vi "temporary CE GUI main.vi"() -> ()   [LabVIEW 2020]
uses:
  Type definitions/CEmeter settings.ctl
  Utilities/Type definitions/Common properties.ctl
  General AC source/Type definitions/AC Source.ctl
  General AC source/Type definitions/AC Source type.ctl
  Utilities/Type definitions/Measurement properties.ctl
panel:
  in  "Settle down after AC source change (s)":dbl=5.0 format="%#_13g"
  in  "AC Source":T1={"AC Source type"=enum."Tektronix AFG3000 series", "VISA"="GPIB0::11::INSTR", "Ref. clock (Hz)"=10000000.0, "status ref"=refnum}
  out "Measurement points":i32
  out "Measurement frequencies":i32[](array[numeric]) caption="List of measurement frequencies"
  in  "Stop freuency (Hz)":i32=7000000 format="%#_7p"
  in  "Step freuency (Hz)":i32=200000 format="%#_7p"
  in  "Starting freuency":i32=1000 format="%#_7p"
  in  "Sampling frequency (Hz)":dbl=10000000.0 format="%#_13p"
  in  "Signal amplitude (V)":dbl=1.0 format="%#_13g"
  in  "AC source status":string
  in  "CEmeter settings":T3={"Common properties"={"Measurement status ref"=refnum, "TWM Status ref"=refnum, "Abort ref"=refnum, "Skip waiting ref"=refnum, "GNU Octave path"=path "C:/Program Files/GNU Octave/Octave-6.2.0/mingw64/bin", "TWM+QWTB path"=path "C:/Users/labina/Desktop/TWM-1.8.7.0-full/octprog", "lvlib path"=path "D:/martin/WAC/WACsw - github/control_software/Filter function meter/external libraries/GOLPI 0.7.3.1 source distribution LV 20.0 32 bit/lv_proc.dll", "TWM pipe"="\\\\.\\pipe\\TWM:server"}, "AC Source"={"AC Source type"=enum."Fluke 5XXX calibrator", "VISA"="", "Ref. clock (Hz)"=0.0, "status ref"=refnum}, "Measurement properties"={"Signal frequencies (Hz)"=[1000.0], "Signal amplitudes (V)"=[0.707], "Sampling frequencies (Hz)"=[10000000.0], "Record lengths (multiples of periods)"=[10000.0], "TWM data directories"=[], "Calculate RMS from samples"=FALSE, "RMS algorithm"="TWM-WFFT"}, "Settle down after AC source change (s)"=1.0} {"Measurement properties"."Record lengths (multiples of periods)" format="%#_3p"; "Measurement properties"."Sampling frequencies (Hz)" format="%#_3p"; "Measurement properties"."Signal amplitudes (V)" format="%#_3p"; "Measurement properties"."Signal frequencies (Hz)" format="%#_3p"}
  in  "Divide frequency by this to\nget number of periods":i32=100
  out "freq / PFI0 A / PFI0 unc(A) / PFI1 A / PFI0 unc(A)":string[][](array[string])
  out "error out":errorcluster
  in  "Skip waiting":bool caption="Abort"
  in  "Abort":bool
  in  "TWM status":string
  in  "mesurement status":string
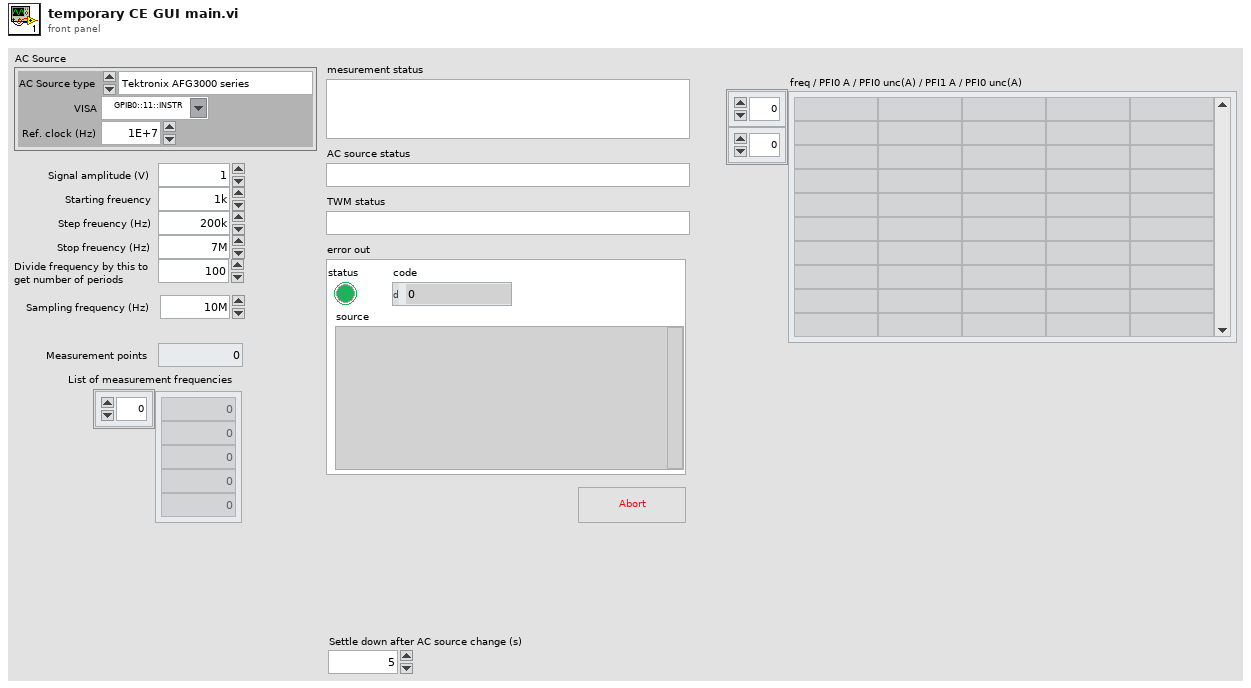
[diagram p1: front panel]
types:
  T1 = typedef "AC Source.ctl" = cluster{"AC Source type":T2, "VISA":refnum<visa-resource-name>, "Ref. clock (Hz)":dbl, "status ref":refnum<vi>}
  T2 = typedef "AC Source type.ctl" = enum16{"Fluke 5XXX calibrator", "Tektronix AFG3000 series", "dummy"}
  T3 = typedef "CEmeter settings.ctl" = cluster{"Common properties":T4, "AC Source":T1, "Measurement properties":T5, "Settle down after AC source change (s)":dbl}
  T4 = typedef "Common properties.ctl" = cluster{"Measurement status ref":refnum<vi>, "TWM Status ref":refnum<vi>, "Abort ref":refnum<vi>, "Skip waiting ref":refnum<vi>, "GNU Octave path":path, "TWM+QWTB path":path, "lvlib path":path, "TWM pipe":string}
  T5 = typedef "Measurement properties.ctl" = cluster{"Signal frequencies (Hz)":dbl[], "Signal amplitudes (V)":dbl[], "Sampling frequencies (Hz)":dbl[], "Record lengths (multiples of periods)":dbl[], "TWM data directories":string[], "Calculate RMS from samples":bool, "RMS algorithm":string}
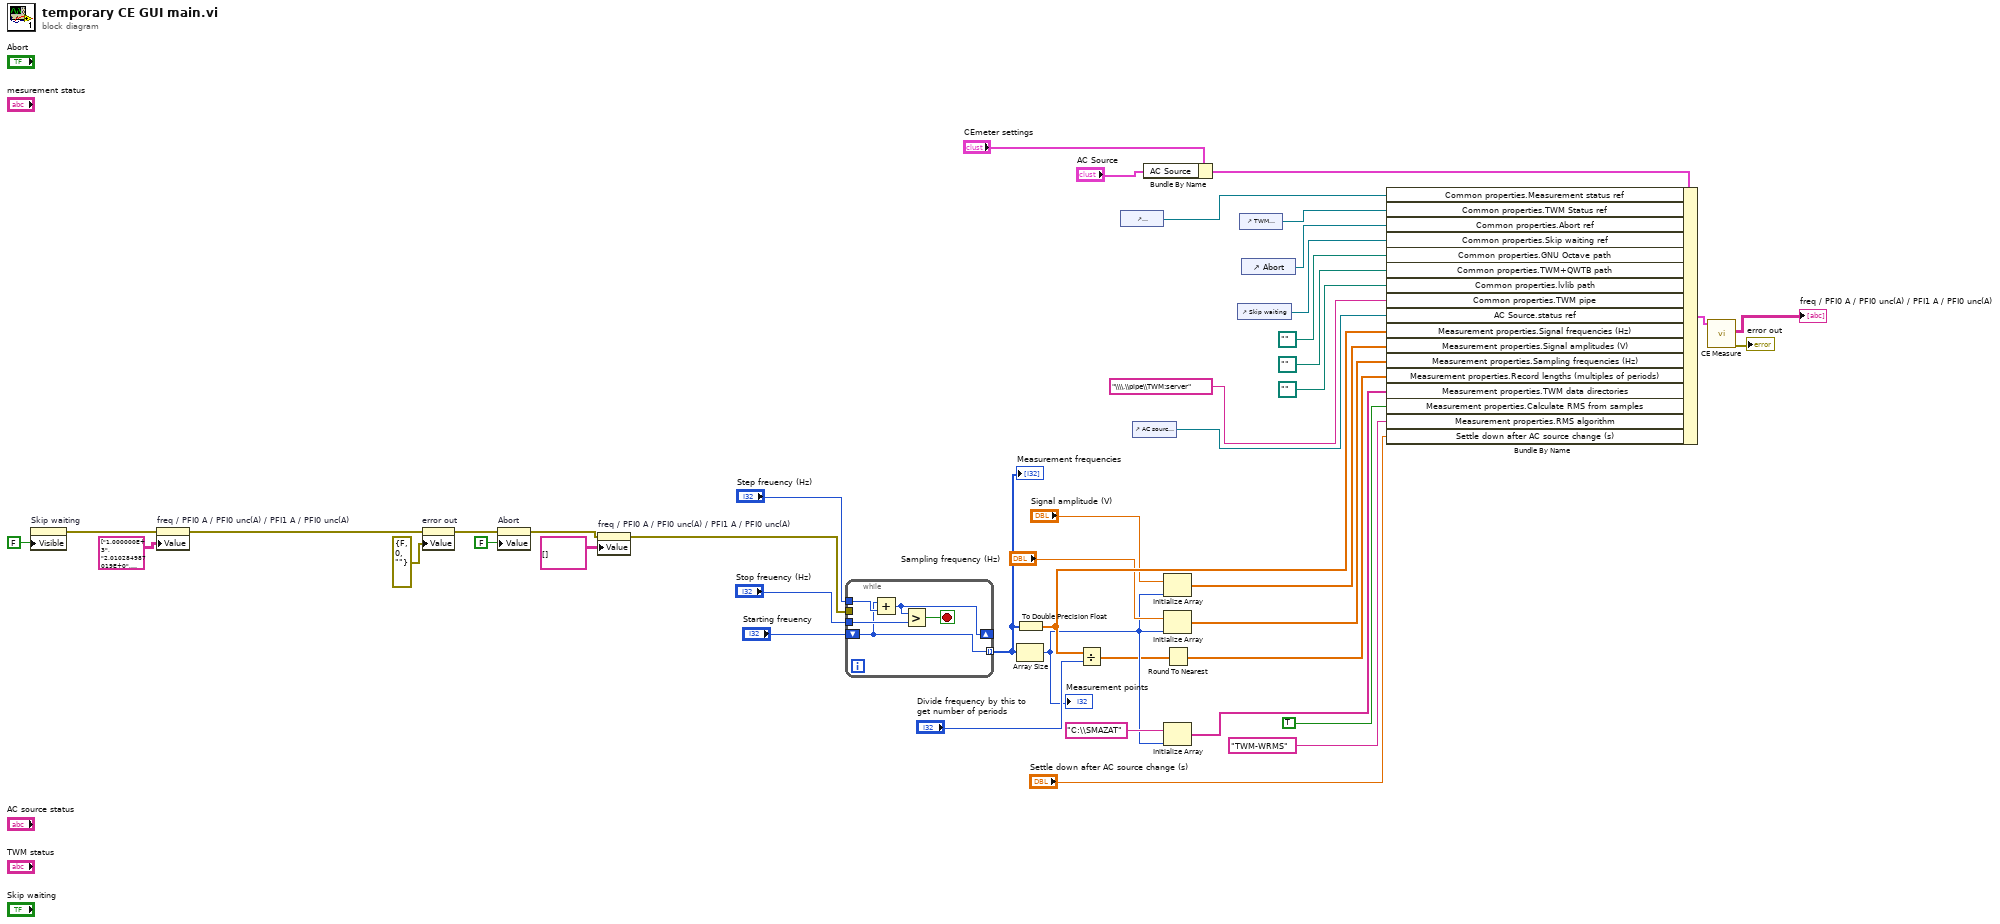
[diagram p0: block diagram]
diagram:
  n1 = property on="Skip waiting" class="Bool (strict)"("Visible"=FALSE) -> (error out=w5:errorcluster)  [unwired: 2 in, 1 out]
  n2 = property on="freq / PFI0 A / PFI0 unc(A) / PFI1 A / PFI0 unc(A)" class="Arr (strict)"(error in=w5, "Value"=string[][] [["1.000000E+3", "2.010284987019E+0", "0.000000000000E+0", "1.811642520698E+0", "0.000000000000E+0"], ["5.100000E+4", "2.013354055463E+0", "0.000000000000E+0", "1.812350667632E+0", "0.000000000000E+0"], ["1.010000E+5", "2.017282793567E+0", "0.000000000000E+0", "1.925150798750E+0", "0.000000000000E+0"], ["1.510000E+5", "2.007397427919E+0", "0.000000000000E+0", "2.013678167807E+0", "0.000000000000E+0"], ["2.010000E+5", "2.003779989445E+0", "0.000000000000E+0", "1.865815841496E+0", "0.000000000000E+0"], ["2.510000E+5", "2.001384962392E+0", "0.000000000000E+0", "1.891179008717E+0", "0.000000000000E+0"], ["3.010000E+5", "1.997468528401E+0", "0.000000000000E+0", "1.906039549706E+0", "0.000000000000E+0"], ["3.510000E+5", "1.996675314976E+0", "0.000000000000E+0", "1.934691135357E+0", "0.000000000000E+0"], ["4.010000E+5", "2.007032360107E+0", "0.000000000000E+0", "1.896204651349E+0", "0.000000000000E+0"], ["4.510000E+5", "1.999368516578E+0", "0.000000000000E+0", "1.950252693112E+0", "0.000000000000E+0"], ["5.010000E+5", "2.007241738713E+0", "0.000000000000E+0", "1.885291684164E+0", "0.000000000000E+0"], ["5.510000E+5", "2.007624589179E+0", "0.000000000000E+0", "1.903361663167E+0", "0.000000000000E+0"], ["6.010000E+5", "2.016149102723E+0", "0.000000000000E+0", "1.845722428962E+0", "0.000000000000E+0"], ["6.510000E+5", "2.017165676146E+0", "0.000000000000E+0", "2.013883211674E+0", "0.000000000000E+0"], ["7.010000E+5", "2.021814939900E+0", "0.000000000000E+0", "1.929805055449E+0", "0.000000000000E+0"], ["7.510000E+5", "2.029974900694E+0", "0.000000000000E+0", "1.864314088932E+0", "0.000000000000E+0"], ["8.010000E+5", "2.028875637501E+0", "0.000000000000E+0", "1.896289161188E+0", "0.000000000000E+0"], ["8.510000E+5", "2.029485375962E+0", "0.000000000000E+0", "1.873795659330E+0", "0.000000000000E+0"], ["9.010000E+5", "2.029221018658E+0", "0.000000000000E+0", "1.835712826595E+0", "0.000000000000E+0"], ["9.510000E+5", "2.022704950204E+0", "0.000000000000E+0", "1.850437083519E+0", "0.000000000000E+0"], ["1.001000E+6", "2.022142263418E+0", "0.000000000000E+0", "1.891579454856E+0", "0.000000000000E+0"], ["1.051000E+6", "2.015557233008E+0", "0.000000000000E+0", "1.851597290198E+0", "0.000000000000E+0"], ["1.101000E+6", "2.019351760745E+0", "0.000000000000E+0", "1.857612683320E+0", "0.000000000000E+0"], ["1.151000E+6", "2.019250353531E+0", "0.000000000000E+0", "1.825346784325E+0", "0.000000000000E+0"], ["1.201000E+6", "2.022136334060E+0", "0.000000000000E+0", "1.886638692802E+0", "0.000000000000E+0"], ["1.251000E+6", "2.014195984626E+0", "0.000000000000E+0", "1.856104171341E+0", "0.000000000000E+0"], ["1.301000E+6", "2.017131895821E+0", "0.000000000000E+0", "1.982884938087E+0", "0.000000000000E+0"], ["1.351000E+6", "2.025822041028E+0", "0.000000000000E+0", "1.863281409219E+0", "0.000000000000E+0"], ["1.401000E+6", "2.036588595132E+0", "0.000000000000E+0", "1.859342585786E+0", "0.000000000000E+0"], ["1.451000E+6", "2.036986754482E+0", "0.000000000000E+0", "1.886647141431E+0", "0.000000000000E+0"], ["1.501000E+6", "2.050390890312E+0", "0.000000000000E+0", "1.882503445845E+0", "0.000000000000E+0"], ["1.551000E+6", "2.047808169123E+0", "0.000000000000E+0", "1.885483086868E+0", "0.000000000000E+0"], ["1.601000E+6", "2.048701317821E+0", "0.000000000000E+0", "1.857872657179E+0", "0.000000000000E+0"], ["1.651000E+6", "2.055672862962E+0", "0.000000000000E+0", "1.890598686585E+0", "0.000000000000E+0"], ["1.701000E+6", "2.051985624670E+0", "0.000000000000E+0", "1.978429584281E+0", "0.000000000000E+0"], ["1.751000E+6", "2.051094118553E+0", "0.000000000000E+0", "1.983173605354E+0", "0.000000000000E+0"], ["1.801000E+6", "2.051849688400E+0", "0.000000000000E+0", "1.881465150776E+0", "0.000000000000E+0"], ["1.851000E+6", "2.053617507568E+0", "0.000000000000E+0", "1.848955914637E+0", "0.000000000000E+0"], ["1.901000E+6", "2.053063941253E+0", "0.000000000000E+0", "1.786170787539E+0", "0.000000000000E+0"], ["1.951000E+6", "2.047171073814E+0", "0.000000000000E+0", "1.790452103112E+0", "0.000000000000E+0"], ["2.001000E+6", "2.056687323747E+0", "0.000000000000E+0", "1.791178165454E+0", "0.000000000000E+0"], ["2.051000E+6", "2.051890239279E+0", "0.000000000000E+0", "1.814018993580E+0", "0.000000000000E+0"], ["2.101000E+6", "2.062729646048E+0", "0.000000000000E+0", "1.813496069392E+0", "0.000000000000E+0"], ["2.151000E+6", "2.062400516961E+0", "0.000000000000E+0", "1.823843473297E+0", "0.000000000000E+0"], ["2.201000E+6", "2.067359801171E+0", "0.000000000000E+0", "1.837206651164E+0", "0.000000000000E+0"], ["2.251000E+6", "2.076697614993E+0", "0.000000000000E+0", "1.745178507572E+0", "0.000000000000E+0"], ["2.301000E+6", "2.086784690967E+0", "0.000000000000E+0", "1.850007877554E+0", "0.000000000000E+0"], ["2.351000E+6", "2.091932995260E+0", "0.000000000000E+0", "1.789696779937E+0", "0.000000000000E+0"], ["2.401000E+6", "2.102613208962E+0", "0.000000000000E+0", "1.771989277419E+0", "0.000000000000E+0"], ["2.451000E+6", "2.100896089553E+0", "0.000000000000E+0", "1.760938349037E+0", "0.000000000000E+0"], ["2.501000E+6", "2.101811129624E+0", "0.000000000000E+0", "1.746517217488E+0", "0.000000000000E+0"], ["2.551000E+6", "2.109958948146E+0", "0.000000000000E+0", "1.806009800328E+0", "0.000000000000E+0"], ["2.601000E+6", "2.103867258930E+0", "0.000000000000E+0", "1.936209323362E+0", "0.000000000000E+0"], ["2.651000E+6", "2.097329185369E+0", "0.000000000000E+0", "1.745223925309E+0", "0.000000000000E+0"], ["2.701000E+6", "2.097383865579E+0", "0.000000000000E+0", "1.805712423638E+0", "0.000000000000E+0"], ["2.751000E+6", "2.103833256344E+0", "0.000000000000E+0", "1.914657159478E+0", "0.000000000000E+0"], ["2.801000E+6", "2.110510288482E+0", "0.000000000000E+0", "1.767984104161E+0", "0.000000000000E+0"], ["2.851000E+6", "2.109456633878E+0", "0.000000000000E+0", "1.728737861971E+0", "0.000000000000E+0"], ["2.901000E+6", "2.111802428017E+0", "0.000000000000E+0", "1.759891673174E+0", "0.000000000000E+0"], ["2.951000E+6", "2.116512445046E+0", "0.000000000000E+0", "1.697987821907E+0", "0.000000000000E+0"], ["3.001000E+6", "2.126290957889E+0", "0.000000000000E+0", "1.744980667078E+0", "0.000000000000E+0"], ["3.051000E+6", "2.137633582331E+0", "0.000000000000E+0", "1.901118500012E+0", "0.000000000000E+0"], ["3.101000E+6", "2.148294114184E+0", "0.000000000000E+0", "1.736920971950E+0", "0.000000000000E+0"], ["3.151000E+6", "2.153176396404E+0", "0.000000000000E+0", "1.729806309026E+0", "0.000000000000E+0"], ["3.201000E+6", "2.164461891598E+0", "0.000000000000E+0", "1.709379570666E+0", "0.000000000000E+0"], ["3.251000E+6", "2.168680484684E+0", "0.000000000000E+0", "1.724619147664E+0", "0.000000000000E+0"], ["3.301000E+6", "2.168354867269E+0", "0.000000000000E+0", "1.738633223405E+0", "0.000000000000E+0"], ["3.351000E+6", "2.172217752521E+0", "0.000000000000E+0", "1.755764122842E+0", "0.000000000000E+0"], ["3.401000E+6", "2.168524779839E+0", "0.000000000000E+0", "1.668117220320E+0", "0.000000000000E+0"], ["3.451000E+6", "2.173816973438E+0", "0.000000000000E+0", "1.698444024296E+0", "0.000000000000E+0"], ["3.501000E+6", "2.164804297899E+0", "0.000000000000E+0", "1.701924040048E+0", "0.000000000000E+0"], ["3.551000E+6", "2.173594436174E+0", "0.000000000000E+0", "1.664711840710E+0", "0.000000000000E+0"], ["3.601000E+6", "2.175936148487E+0", "0.000000000000E+0", "1.698355899553E+0", "0.000000000000E+0"], ["3.651000E+6", "2.184032250860E+0", "0.000000000000E+0", "1.702058849561E+0", "0.000000000000E+0"], ["3.701000E+6", "2.191709077473E+0", "0.000000000000E+0", "1.681773067551E+0", "0.000000000000E+0"], ["3.751000E+6", "2.211264701181E+0", "0.000000000000E+0", "1.634852276923E+0", "0.000000000000E+0"], ["3.801000E+6", "2.214808306204E+0", "0.000000000000E+0", "1.700091687763E+0", "0.000000000000E+0"], ["3.851000E+6", "2.229507643000E+0", "0.000000000000E+0", "1.845430537732E+0", "0.000000000000E+0"], ["3.901000E+6", "2.241741505692E+0", "0.000000000000E+0", "1.677024087213E+0", "0.000000000000E+0"], ["3.951000E+6", "2.245951599543E+0", "0.000000000000E+0", "1.664671147239E+0", "0.000000000000E+0"], ["4.001000E+6", "2.226008559815E+0", "0.000000000000E+0", "1.639802119328E+0", "0.000000000000E+0"], ["4.051000E+6", "2.200489575248E+0", "0.000000000000E+0", "1.602034034675E+0", "0.000000000000E+0"], ["4.101000E+6", "2.159605503881E+0", "0.000000000000E+0", "1.583503289306E+0", "0.000000000000E+0"], ["4.151000E+6", "2.098767874496E+0", "0.000000000000E+0", "1.520924381070E+0", "0.000000000000E+0"], ["4.201000E+6", "2.004624328108E+0", "0.000000000000E+0", "1.446548539299E+0", "0.000000000000E+0"], ["4.251000E+6", "1.898920288350E+0", "0.000000000000E+0", "1.497998781546E+0", "0.000000000000E+0"], ["4.301000E+6", "1.769735919476E+0", "0.000000000000E+0", "1.269627080842E+0", "0.000000000000E+0"], ["4.351000E+6", "1.622205310245E+0", "0.000000000000E+0", "1.201115226842E+0", "0.000000000000E+0"], ["4.401000E+6", "1.455230415572E+0", "0.000000000000E+0", "1.128480473830E+0", "0.000000000000E+0"], ["4.451000E+6", "1.279947598767E+0", "0.000000000000E+0", "9.410900285284E-1", "0.000000000000E+0"], ["4.501000E+6", "1.101639634592E+0", "0.000000000000E+0", "8.939591050168E-1", "0.000000000000E+0"]] ("freq / PFI0 A / PFI0 unc(A) / PFI1 A / PFI0 unc(A)")) -> (error out=w4:errorcluster)  [unwired: 1 in, 1 out]
  n3 = property on="error out" class="Clust (strict)"(error in=w4, "Value"=errorcluster {"status"=FALSE, "code"=0, "source"=""}) -> (error out=w3:errorcluster)  [unwired: 1 in, 1 out]
  n4 = property on="Abort" class="Bool (strict)"(error in=w3, "Value"=FALSE ("Abort")) -> (error out=w2:errorcluster)  [unwired: 1 in, 1 out]
  n5 = property on="freq / PFI0 A / PFI0 unc(A) / PFI1 A / PFI0 unc(A)" class="Arr (strict)"(error in=w2, "Value"=string[][] [] ("freq / PFI0 A / PFI0 unc(A) / PFI1 A / PFI0 unc(A)")) -> (error out=w1:errorcluster)  [unwired: 1 in, 1 out]
  n6 = while {
    tunnel: "Step freuency (Hz)" -> [w48]
    tunnel: "Stop freuency (Hz)" -> [w47]
    shift-right: [w46] -> _
    shift-left: "Starting freuency" -> [w44]
    tunnel: [w44] -> w19 mode=indexing
    tunnel: w1 -> [_]
    stop <- w45 stop-if-true
    n7 = Add(x=w44, y=w48) -> (x+y=w46:i32)
    n8 = Greater?(x=w46, y=w47) -> (0:w45:bool)
  }
  "Measurement frequencies" <- w19
  n9 = Array Size(array=w19) -> (size(s)=w17:i32)
  "Measurement points" <- w17
  n10 = To Double Precision Float(number=w19) -> (double precision float=w29:dbl[])
  n11 = Divide(x=w29, y="Divide frequency by this to\nget number of periods") -> (x/y=w12:dbl[])
  n12 = control-ref of="mesurement status"() -> (w40:refnum<vi>)
  n13 = control-ref of="AC source status"() -> (w27:refnum<vi>)
  n14 = Bundle By Name(cluster="CEmeter settings", "AC Source"="AC Source") -> (w13:T3)
  n15 = Initialize Array("Signal amplitude (V)", w17) -> (w22:dbl[])
  n16 = Initialize Array("Sampling frequency (Hz)", w17) -> (w20:dbl[])
  n17 = Round To Nearest(number=w12) -> (nearest integer value=w11:dbl[])
  n18 = Initialize Array("C:\\SMAZAT" ("Measurement properties.Algorithm"), w17) -> (w16:string[])
  n19 = control-ref of="Skip waiting"() -> (w37:refnum<vi>)
  n20 = control-ref of="TWM status"() -> (w39:refnum<vi>)
  n21 = control-ref of="Abort"() -> (w38:refnum<vi>)
  n22 = Bundle By Name(cluster=w13, "Common properties.Measurement status ref"=w40, "Common properties.TWM Status ref"=w39, "Common properties.Abort ref"=w38, "Common properties.Skip waiting ref"=w37, "Common properties.GNU Octave path"=path "", "Common properties.TWM+QWTB path"=path "", "Common properties.lvlib path"=path "", "Common properties.TWM pipe"="\\\\.\\pipe\\TWM:server" ("TWM pipe"), "AC Source.status ref"=w27, "Measurement properties.Signal frequencies (Hz)"=w29, "Measurement properties.Signal amplitudes (V)"=w22, "Measurement properties.Sampling frequencies (Hz)"=w20, "Measurement properties.Record lengths (multiples of periods)"=w11, "Measurement properties.TWM data directories"=w16, "Measurement properties.Calculate RMS from samples"=TRUE, "Measurement properties.RMS algorithm"="TWM-WRMS" ("Measurement properties.Algorithm"), "Settle down after AC source change (s)"="Settle down after AC source change (s)") -> (w28:T3)
  n23 = call "CE Measure.vi"("CEmeter settings"=w28) -> ("error out"=→"error out":errorcluster, "TWM results"=→"freq / PFI0 A / PFI0 unc(A) / PFI1 A / PFI0 unc(A)":string[][])  [unwired: 9 in]
